vi "Process.vi"(11 "obj":refnum<class "SciWare_ByRefActiveObj_V1.0.0.lvclass">) -> ()   [LabVIEW 2009, in "SciWare_ByRefActiveObj_V1.0.0.lvclass"]
doc: "Active object process.\n\nBSD License (http://www.opensource.org/licenses/bsd-license.php)"
uses:
  SciWare_ByRefActiveObj_V1.0.0.lvclass
  SciWare_ByRefActiveObj_V1.0.0.lvclass/SciWare_ByRefActiveObj_V1.0.0.ctl
panel:
  # "BSD License (http://www.opensource.org/licenses/bsd-license.php)"
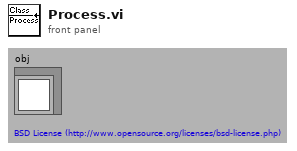
[diagram p1: front panel]
types:
  T1 = typedef "SciWare_ByRefActiveObj_V1.0.0.lvclass/DataRef.ctl" = refnum<data-value>
  T2 = typedef "SciWare_ByRefActiveObj_V1.0.0.lvclass/CmdQueueRef.ctl" = refnum<queue>
  T3 = typedef "SciWare_ByRefActiveObj_V1.0.0.lvclass/CmdQueueType.ctl" = string
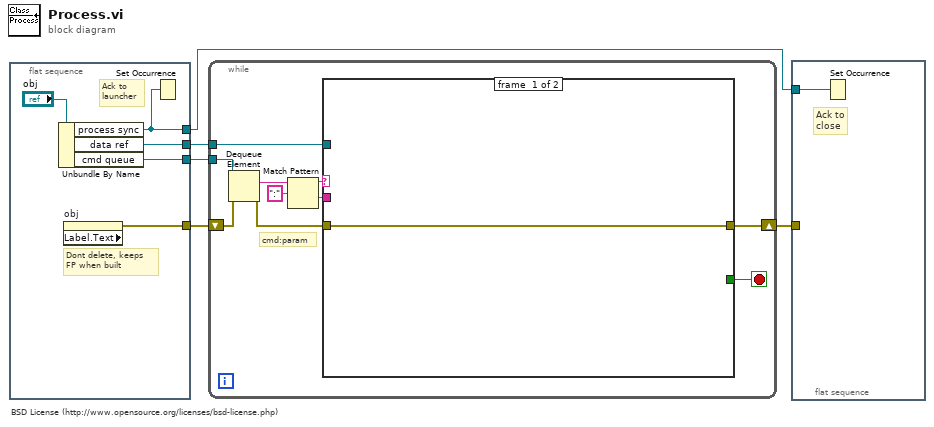
[diagram p0: block diagram]
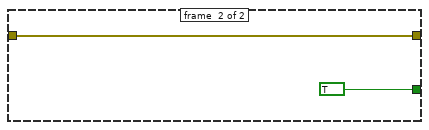
[diagram p2: hidden frame]
diagram:
  # "BSD License (http://www.opensource.org/licenses/bsd-license.php)"
  n1 = flat-sequence {
    tunnel: [w9] -> w5
    tunnel: [w8] -> w3
    tunnel: [w6] -> w2
    tunnel: [w7] -> w1
    frame #0 {
      # "Ack to\nlauncher"
      # "Dont delete, keeps\nFP when built"
      n2 = Unbundle By Name("obj") -> ("process sync"=w7:refnum<k4>, "data ref"=w8:T1, "cmd queue"=w9:T2)
      n3 = property on="obj" class="LVClassControl (strict)" props=["Label", "Text"]() -> (error out=w6:errorcluster)  [unwired: 2 in, 2 out]
      n4 = Set Occurrence(w7) -> ()
    }
  }
  n5 = while {
    tunnel: w5 -> [w20]
    shift-right: [w17] -> w4
    shift-left: w2 -> [w19]
    tunnel: w3 -> [w15]
    stop <- w16 stop-if-true
    # "cmd:param"
    n6 = Dequeue Element(queue=w20, error in (no error)=w19) -> (element=w14:T3, error out=w18:errorcluster)  [unwired: 1 in, 2 out]
    n7 = Match Pattern(string=w14, regular expression=":") -> (before substring=w13:T3, after substring=w11:T3)  [unwired: 1 in, 2 out]
    n8 = case shown="\"shutdown\"" w13 {
      tunnel: [w21 w23] -> w17
      tunnel: w18 -> [w21 w23]
      tunnel: [_ TRUE] -> w16
      tunnel: w15 -> [_ _]
      tunnel: w11 -> [_ _]
      frame #0 {
      }
      frame #1 {
      }
    }
  }
  n9 = flat-sequence {
    tunnel: w4 -> [_]
    tunnel: w1 -> [w24]
    frame #0 {
      # "Ack to\nclose"
      n10 = Set Occurrence(w24) -> ()
    }
  }
